vi "ex13.vi"() -> ()   [LabVIEW 2019]
panel:
  in  "y":dbl
  out "x+y":dbl
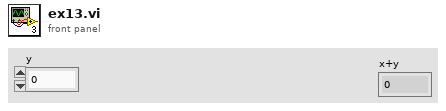
[diagram p1: front panel]
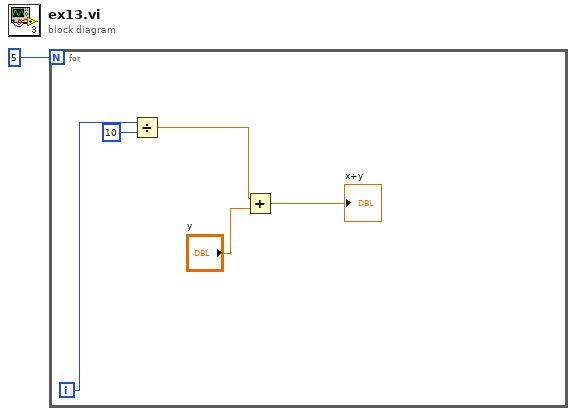
[diagram p0: block diagram]
diagram:
  n1 = for {
    N: 5 -> [_]
    i -> [w3]
    n2 = Divide(x=w3, y=10) -> (x/y=w4:dbl)
    n3 = Add(x=w4, y="y") -> (x+y=→"x+y":dbl)
  }
